vi "Number to Column Letter.vi"(11 "Number":u32) -> (3 "Letter":string)   [LabVIEW 2021, in "Open Xml.lvlib"]
uses:
  Open Xml.lvlib
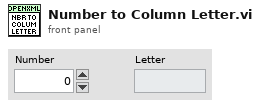
[diagram p1: front panel]
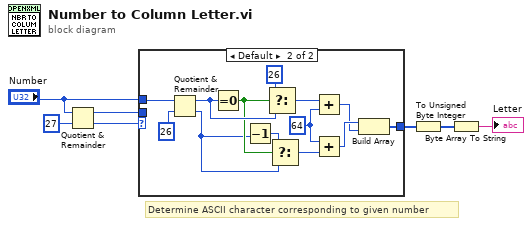
[diagram p0: block diagram]
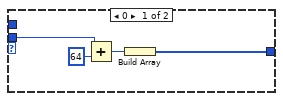
[diagram p2: hidden frame]
diagram:
  # "Determine ASCII character corresponding to given number"
  n1 = Quotient & Remainder(x="Number", y=27) -> (x-y*floor(x/y)=w6:u32, floor(x/y)=w3:u32)
  n2 = case shown="Default" w3 {
    tunnel: "Number" -> [_ w12]
    tunnel: w6 -> [w11 _]
    tunnel: [w10 w14] -> w5
    frame 0 {
      n3 = Add(x=w11, y=64) -> (x+y=w8:u32)
      n4 = Build Array(w8) -> (w10:u32[])
    }
    frame Default {
      w13 = 64
      n5 = Quotient & Remainder(x=w12, y=26) -> (x-y*floor(x/y)=w22:u32, floor(x/y)=w19:u32)
      n6 = Equal To 0?(x=w22) -> (x = 0?=w20:bool)
      n7 = Decrement(x=w19) -> (x-1=w21:u32)
      n8 = Select(t=26, s=w20, f=w22) -> (s? t:f=w18:u32)
      n9 = Select(t=w21, s=w20, f=w19) -> (s? t:f=w17:u32)
      n10 = Add(x=w18, y=w13) -> (x+y=w15:u32)
      n11 = Add(x=w13, y=w17) -> (x+y=w16:u32)
      n12 = Build Array(w16, w15) -> (w14:u32[])
    }
  }
  n13 = To Unsigned Byte Integer(number=w5) -> (unsigned 8bit integer=w4:u8[])
  n14 = Byte Array To String(unsigned byte array=w4) -> (string=→"Letter":string)
